vi "getEventHeartbeat.vi"(8 "error in (no error)":errorcluster, 11 "SALCommunicatorTC in":refnum<class "SALCommunicatorTC.lvclass">) -> (0 "error out":errorcluster, 1 "Heartbeat":bool, 2 "function return":i32, 3 "SALCommunicatorTC out":refnum<class "SALCommunicatorTC.lvclass">)   [LabVIEW 2016, in "SALCommunicatorTC.lvclass"]
uses:
  SALCommunicatorTC.lvclass
  ts_sallv_exa/SALLV_EXA.lvlib
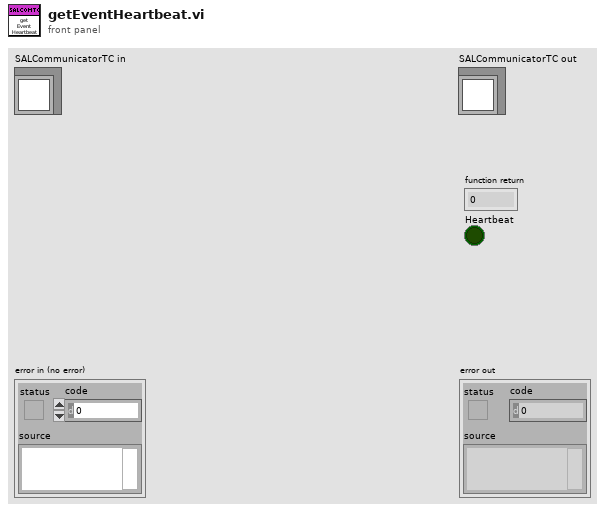
[diagram p1: front panel]
types:
  T1 = typedef "SALLV_EXA.lvlib/logevent_Heartbeat.ctl" = cluster{"Heartbeat":bool, "priority":i32}
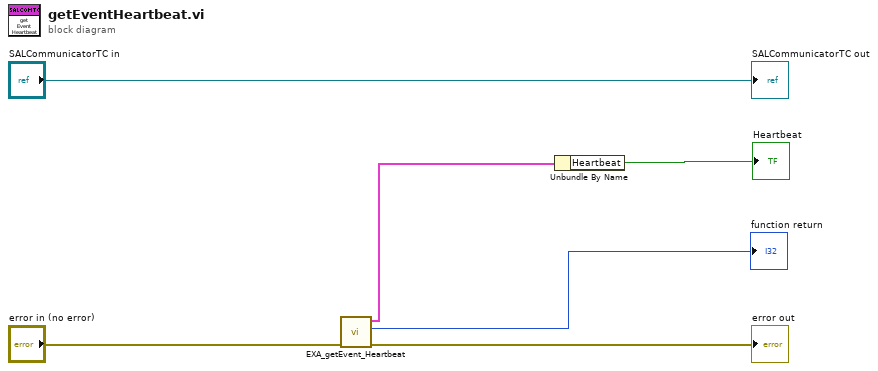
[diagram p0: block diagram]
diagram:
  n1 = call "EXA_getEvent_Heartbeat.vi"("error in (no error)"="error in (no error)") -> ("error out"=→"error out":errorcluster, "function return"=→"function return":i32, "logevent_Heartbeat_Ctl out"=w2:T1)  [unwired: 8 in]
  n2 = Unbundle By Name(w2) -> ("Heartbeat"=→"Heartbeat":bool)
  "SALCommunicatorTC out" <- "SALCommunicatorTC in"
